vi "_PC_Daemon_RecipeEditor.vi"(5 "eng_mode_str":refnum<vi>, 8 "error in (no error)":errorcluster, 11 "Network\nstream":refnum<vi>) -> (0 "error out":errorcluster)   [LabVIEW 2018]
uses:
  System.Windows.Forms
  winForms/winForms editorType.ctl
  <vilib>/Utility/miscctls.llb/LVRowAndColumnTypeDef.ctl
  C:/ATI_MS_InstrumentControl/dll/ScintillaNET.dll
  dll/ScintillaNET.dll
  PublicSubVI/Ctl/RegistyFunc.ctl
  RecipeEditorPython/subVI/getScriptInfo.ctl
  PublicSubVI/Class/DataXML/DataXML dataType.ctl
  RecipeEditor/MSEncoder/MSEncoder.lvclass
  PublicSubVI/Class/QMH/QMH.lvclass
  PublicSubVI/Class/DataXML/DataXML.lvclass
panel:
  in  "SaveScript":bool
  in  "SaveScript_new":bool
  in  "open script":bool caption="OpenScript"
  in  "searchText":string
  in  "checkScript":bool
  in  "save_method":bool
  in  "applyScript":bool caption="apply_script"
  in  "help":bool caption="helpBtn"
  out "file path":string
  in  "script":refnum<k24>(container)
  in  "Parameter Tab":enum32{"User Parameter", "Instrument Parameter"}(tab)
  in  "user param table":string[][](table)
  in  "instr param table":string[][](table)
  in  "Dialogue":i32(listbox)=-1
  in  "stop":bool
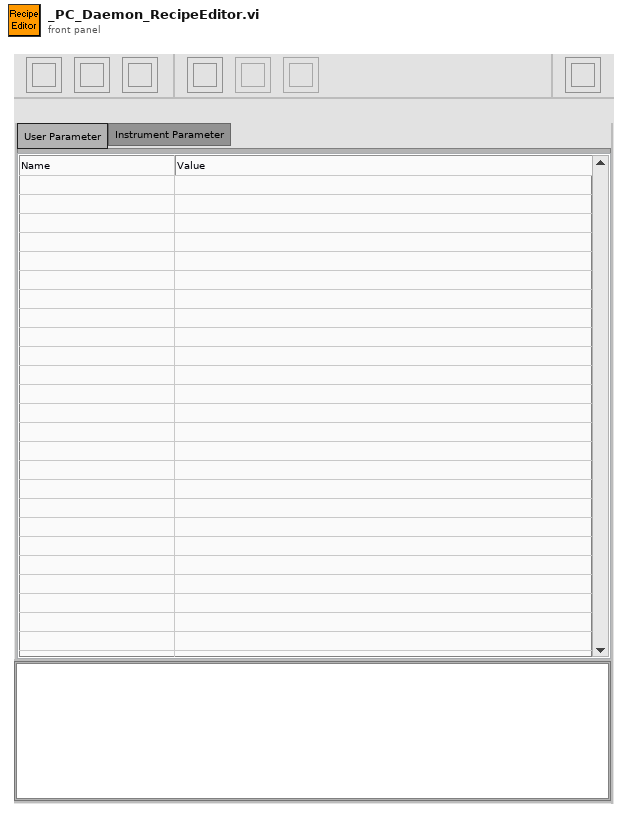
[diagram p1: front panel]
types:
  T1 = enum8{"Enabled", "Disabled", "Disabled and Grayed Out"}
  T2 = typedef "winForms editorType.ctl" = enum16{"Recipe", "SigProc", "Editor"}
  T3 = enum32{"Invalid", "Default", "Floating", "Floating/Auto-Hide", "Modal"}
  T4 = typedef "LVRowAndColumnTypeDef.ctl" = cluster{"Row":i32, "Column":i32}
  T5 = enum32{"Invalid", "Standard", "Closed", "Hidden", "Minimized", "Maximized"}
  T6 = enum16{"No Scaling", "Scale All Objects", "Scale Single Object"}
  T7 = typedef "LVRectTypeDef.ctl" = cluster{"Left":i16, "Top":i16, "Right":i16, "Bottom":i16}
  T8 = typedef "getScriptInfo.ctl" = enum16{"userEditor", "userParam", "instrParam", "sourcePath", "sourceTimeStamp", "versionInfo"}
  T9 = enum16{"open", "replace", "create", "open or create", "replace or create", "replace or create with confirmation"}
  T10 = typedef "DataXML dataType.ctl" = enum16{"Instrument", "UserInterface", "SampleType", "UserDefined"}
  T11 = cluster{"ProcessCodes":u64[], "WfmCodes":u64[], "Signal Remarks":cluster{"mzID":u64, "SignalInfo":cluster{"Label":string, "dt":dbl, "Length":u32, "RefVolt":dbl, "mzTable":cluster{"t":dbl[], "mz":dbl[], "beta":dbl[]}}[]}, "scriptCode":string}
  T12 = typedef "eventvkey.ctl" = enum16{"ASCII", "Enter", "Return", "Shift", "Ctrl", "Alt", "Cmd", "Opt", "Caps", "NumLock", "Clear", "Break", "Up", "Down", "Left", "Right", "Insert", "Delete", "Home", "End", "PageUp", "PageDown", "Escape", "Help", "Pause", "ScrollLock", "F1", "F2", "F3", "F4", "F5", "F6", "F7", "F8", "F9", "F10", "F11", "F12", "F13", "F14", "F15", "F16", "F17", "F18", "F19", "F20", "F21", "F22", "F23", "F24", "Play", "VolumeUp", "VolumeDown", "Mute", "Two Byte Char"}
  T13 = typedef "RegistyFunc.ctl" = enum16{"None", "FileAutoSave", "FileNoise", "FileSN", "ExeStatu", "WorkFolderPath", "MethodPath", "AVGItem", "LoopItem", "AutoRun", "BGColor", "LineColor", "LineWidth", "XGrid", "YGrid", "DeviceRefnum"}
  T14 = typedef "LVPoint32TypeDef.ctl" = cluster{"Horizontal":i32, "Vertical":i32}
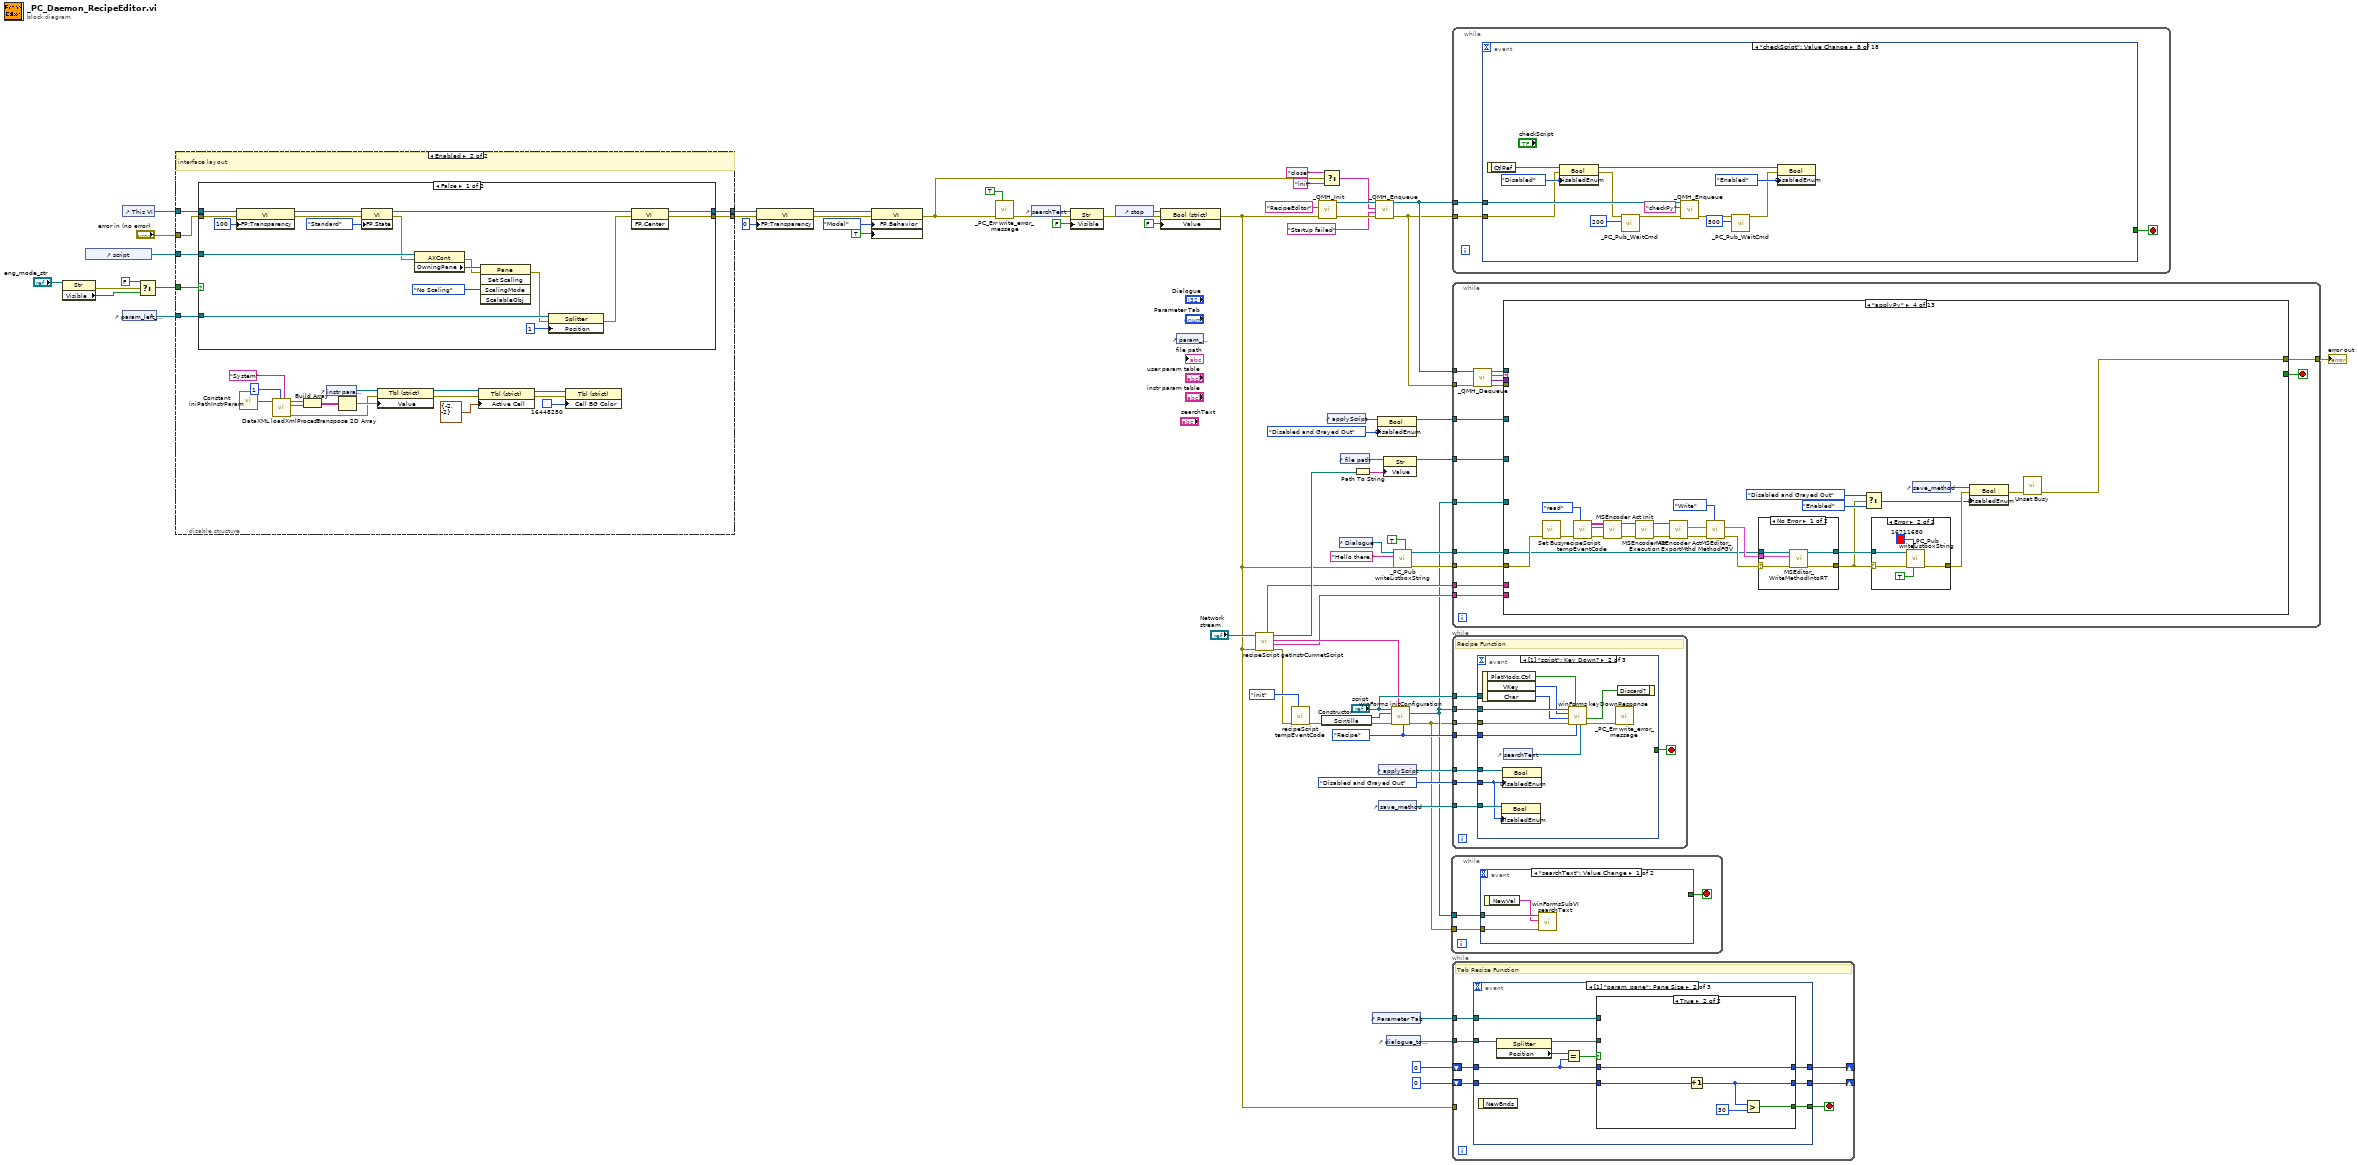
[diagram p0: block diagram]
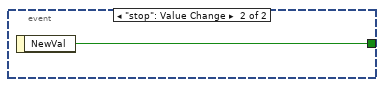
[diagram p2: hidden frame]
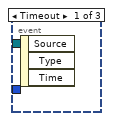
[diagram p3: hidden frame]
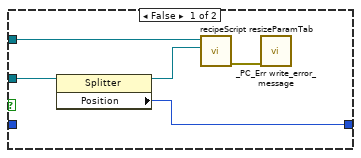
[diagram p4: hidden frame]
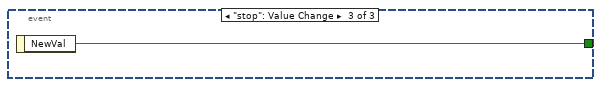
[diagram p5: hidden frame]
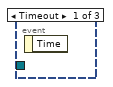
[diagram p6: hidden frame]
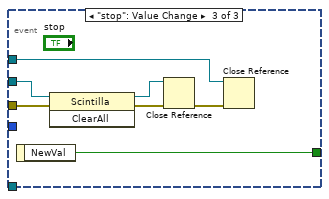
[diagram p7: hidden frame]
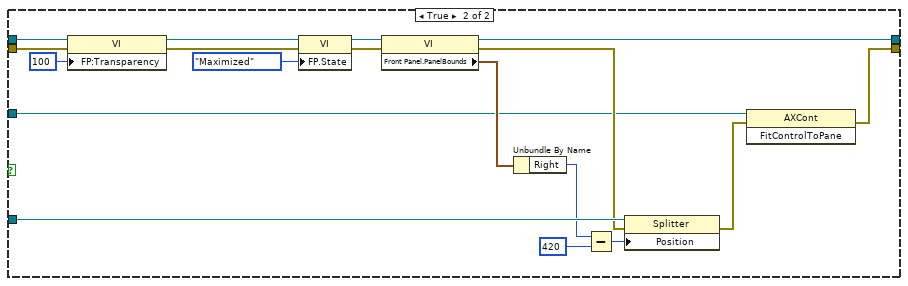
[diagram p9: hidden frame]
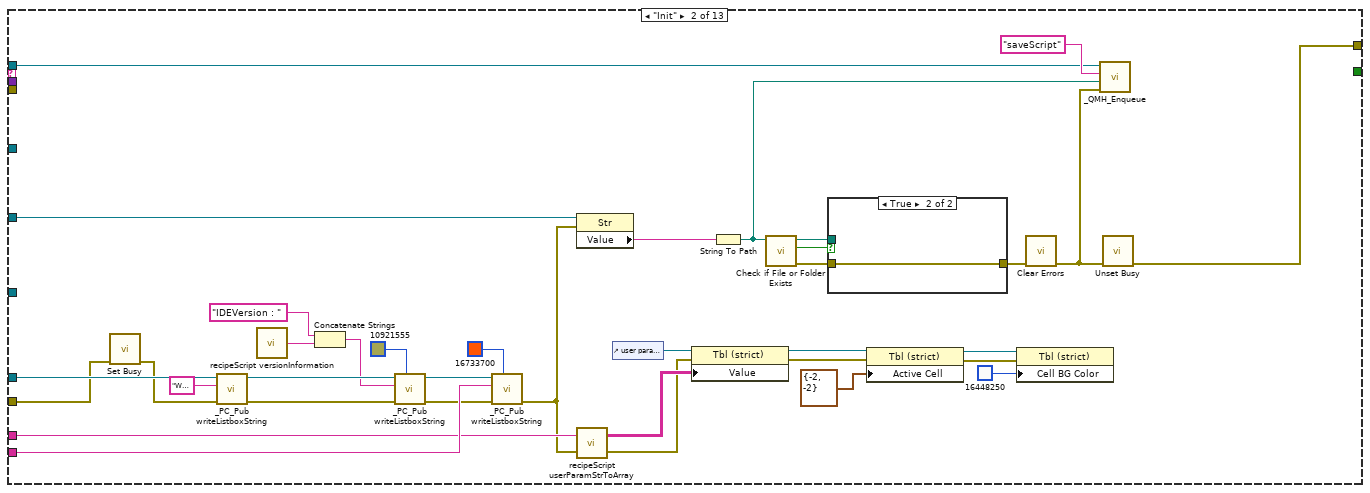
[diagram p11: hidden frame]
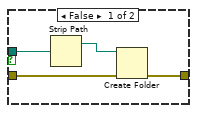
[diagram p12: hidden frame]
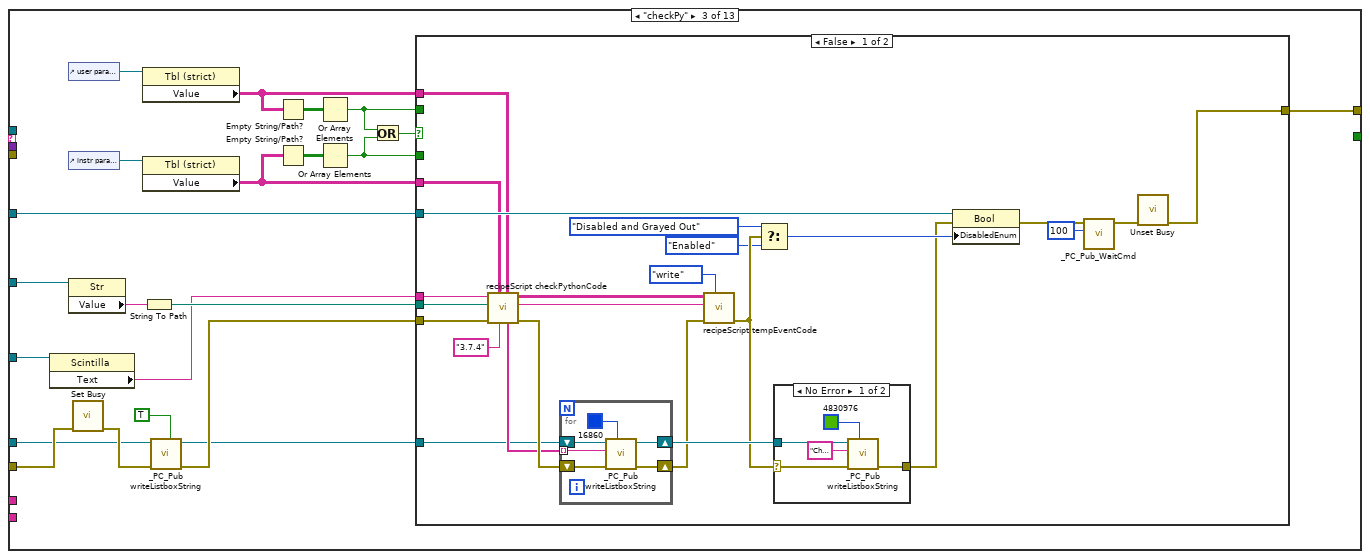
[diagram p13: hidden frame]
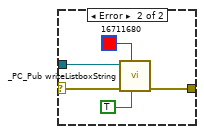
[diagram p14: hidden frame]
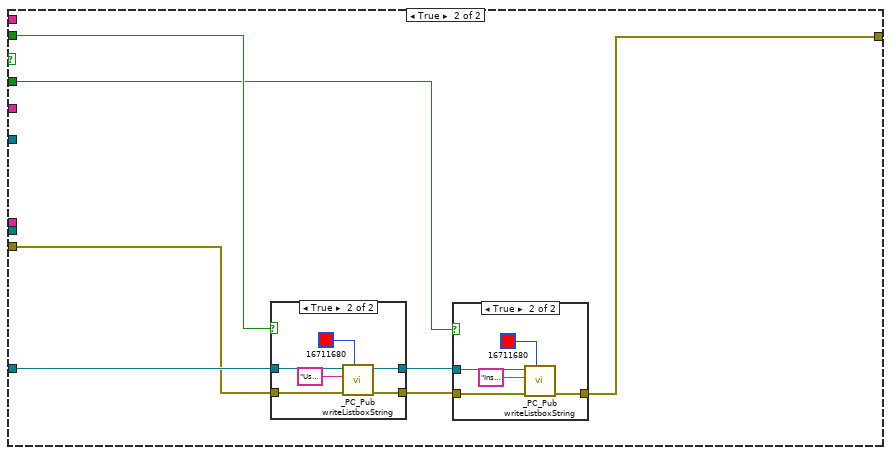
[diagram p15: hidden frame]
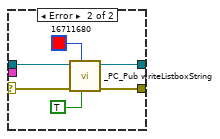
[diagram p19: hidden frame]
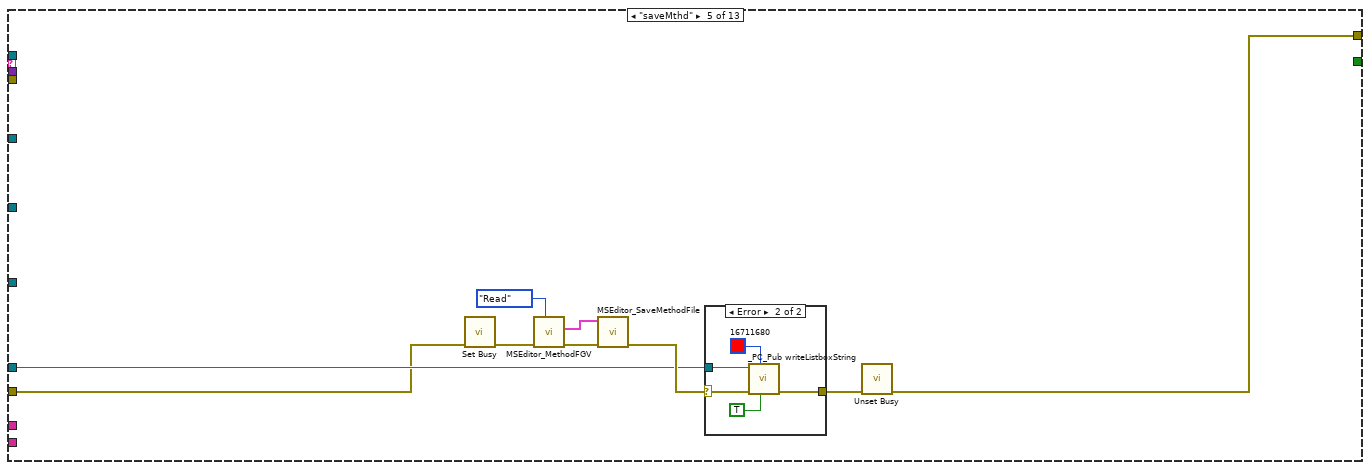
[diagram p20: hidden frame]
diagram:
  w15 = winForms_editorType."Recipe" ("editorType")
  n1 = property class="Str"(reference="eng_mode_str") -> (error out=w40:errorcluster, "Visible"=w39:bool)  [unwired: 1 in, 1 out]
  n2 = control-ref of="script"() -> (w36:refnum<vi>)
  n3 = control-ref of="param_left_spl"() -> (w64:refnum<vi>)
  n4 = control-ref of="This VI"() -> (w43:refnum<vi>)
  n5 = Select(t=FALSE, s=w40, f=w39) -> (s? t:f=w37:bool)
  n6 = disable-structure shown="Enabled" {
    disable-tunnel: w37 -> [_ w68]
    disable-tunnel: "error in (no error)" -> [_ w85]
    disable-tunnel: w43 -> [_ w87]
    disable-tunnel: [_ w86] -> w65
    disable-tunnel: w64 -> [_ w89]
    disable-tunnel: w36 -> [_ w88]
    disable-tunnel: [_ w69] -> w41
    frame Disabled {
    }
    frame Enabled {
      # "interface layout"
      n7 = case shown="False" w68 {
        tunnel: w89 -> [w107 w125]
        tunnel: w88 -> [w102 w114]
        tunnel: w87 -> [w99 w112]
        tunnel: [w90 w119] -> w86
        tunnel: [w91 w108] -> w69
        tunnel: w85 -> [w98 w111]
        frame False {
          n8 = property class="VI"(reference=w99, error in=w98, "FP:Transparency"=u8 100 ("Front Panel Window:Transparency")) -> (reference out=w96:refnum<vi>, error out=w95:errorcluster)
          n9 = property class="VI"(reference=w96, error in=w95, "FP.State"=T5."Standard" ("Front Panel Window:State")) -> (reference out=w93:refnum<vi>, error out=w94:errorcluster)
          n10 = property class="AXCont"(reference=w102, error in=w94) -> (error out=w103:errorcluster, "OwningPane"=w105:refnum<vi>)  [unwired: 1 out]
          n11 = invoke class="Pane" method="Set Scaling"(reference=w105, error in=w103, "ScalingMode"=T6."No Scaling" ("Scaling Mode")) -> (error out=w101:errorcluster)  [unwired: 2 in, 4 out]
          n12 = property class="Splitter"(reference=w107, error in=w101, "Position"=1 ("Splitter Position")) -> (error out=w92:errorcluster)  [unwired: 1 out]
          n13 = invoke class="VI" method="FP.Center"(reference=w93, error in=w92) -> (reference out=w90:refnum<vi>, error out=w91:errorcluster)  [unwired: 1 in, 1 out]
        }
        frame True {
          n14 = property class="VI"(reference=w112, error in=w111, "FP:Transparency"=u8 100 ("Front Panel Window:Transparency")) -> (reference out=w110:refnum<vi>, error out=w109:errorcluster)
          n15 = property class="VI"(reference=w110, error in=w109, "FP.State"=T5."Maximized" ("Front Panel Window:State")) -> (reference out=w122:refnum<vi>, error out=w121:errorcluster)
          n16 = property class="VI"(reference=w122, error in=w121) -> (reference out=w119:refnum<vi>, error out=w120:errorcluster, "Front Panel.PanelBounds"=w118:T7)
          n17 = Unbundle By Name(w118) -> ("Right"=w117:i16)
          n18 = Subtract(x=w117, y=i16 420) -> (x-y=w115:i16)
          n19 = property class="Splitter"(reference=w125, error in=w120, "Position"=w115) -> (error out=w124:errorcluster)  [unwired: 1 out]
          n20 = invoke class="AXCont" method="FitControlToPane"(reference=w114, error in=w124) -> (error out=w108:errorcluster)  [unwired: 1 in, 2 out]
        }
      }
      n21 = call "Constant iniPathInstrParam.vi"() -> ("appended path"=w81:path)
      n22 = call "DataXML loadXmlProcess.vi"("target name"="System", "level"=u8 1, "xml_data_path"=w81) -> ("error IO"=w70:errorcluster, "value"=w83:string[], "name"=w82:string[])  [unwired: 5 in, 1 out]
      n23 = Build Array(w82, w83) -> (w84:string[][])
      n24 = control-ref of="instr param table"() -> (w74:refnum<vi>)
      n25 = Transpose 2D Array(2D array=w84) -> (transposed array=w73:string[][])
      n26 = property class="Tbl (strict)"(reference=w74, error in=w70, "Value"=w73) -> (reference out=w75:refnum<vi>, error out=w76:errorcluster)
      n27 = property class="Tbl (strict)"(reference=w75, error in=w76, "Active Cell"=T4 {"Row"=-2, "Column"=-2} ("Active Cell:Active Cell")) -> (reference out=w77:refnum<vi>, error out=w78:errorcluster)
      n28 = property class="Tbl (strict)"(reference=w77, error in=w78, "Cell BG Color"=u32 16448250) -> ()  [unwired: 2 out]
    }
  }
  n29 = property class="VI"(reference=w65, error in=w41, "FP:Transparency"=u8 0 ("Front Panel Window:Transparency")) -> (reference out=w57:refnum<vi>, error out=w58:errorcluster)
  n30 = property class="VI"(reference=w57, error in=w58, "FP.Behavior"=T3."Modal" ("Front Panel Window:Behavior"), "Front Panel.IsFrontmost"=TRUE ("Front Panel Window:Is Frontmost")) -> (error out=w28:errorcluster)  [unwired: 1 out]
  n31 = call "_PC_Err write_error_message.vi"("show msg( T )"=TRUE, "error in"=w28) -> ("error out"=w5:errorcluster)  [unwired: 9 in]
  n32 = control-ref of="searchText"() -> (w6:refnum<vi>)
  n33 = property class="Str"(reference=w6, error in=w5, "Visible"=FALSE) -> (error out=w4:errorcluster)  [unwired: 1 out]
  n34 = control-ref of="stop"() -> (w35:refnum<vi>)
  n35 = property class="Bool (strict)"(reference=w35, error in=w4, "Value"=FALSE) -> (error out=w17:errorcluster)  [unwired: 1 out]
  n36 = control-ref of="param_pane"() -> ()  [unwired: 1 out]
  n37 = call "recipeScript getInstrCurrnetScript.vi"("error in (no error)"=w17, "Network\nstream"="Network\nstream") -> ("error out"=w13:errorcluster, "versionInfo"=w8:string, "initScriptCode"=w16:string, "initFilePath"=w19:path, "userParam"=w7:string)  [unwired: 5 in]
  n38 = call "recipeScript tempEventCode.vi"("type"=enum16{"init", "write", "read"}."init", "error in (no error)"=w13) -> ("error out"=w12:errorcluster)  [unwired: 7 in, 2 out]
  n39 = call "_QMH_Init.vi"("error in (no error)"=w17, "name (unnamed)"="RecipeEditor") -> ("error out"=w62:errorcluster, "QMH out"=w63:refnum<class "QMH.lvclass">)  [unwired: 8 in]
  n40 = constructor class="Scintilla"(error in=w12) -> (reference out=w25:refnum<k24>, error out=w24:errorcluster)  [unwired: 2 in, 1 out]
  n41 = Select(t="close" ("Msg"), s=w28, f="init" ("Msg")) -> (s? t:f=w51:string)
  n42 = control-ref of="applyScript"() -> (w46:refnum<vi>)
  n43 = control-ref of="Dialogue"() -> (w55:refnum<vi>)
  n44 = control-ref of="file path"() -> (w21:refnum<vi>)
  n45 = Path To String(path=w19) -> (string=w18:string)
  n46 = control-ref of="Parameter Tab"() -> (w32:refnum<vi>)
  n47 = call "_QMH_Enqueue.vi"("error in (no error)"=w62, "Data"="Startup failed", "Msg"=w51, "QMH in"=w63) -> ("error out"=w48:errorcluster, "QMH out"=w61:refnum<class "QMH.lvclass">)  [unwired: 6 in]
  n48 = property class="Bool"(reference=w46, "DisabledEnum"=T1."Disabled and Grayed Out" ("Disabled")) -> (reference out=w45:refnum<vi>)  [unwired: 1 in, 1 out]
  n49 = control-ref of="applyScript"() -> (w11:refnum<vi>)
  n50 = control-ref of="save_method"() -> (w9:refnum<vi>)
  n51 = property class="Str"(reference=w21, "Value"=w18) -> (reference out=w20:refnum<vi>)  [unwired: 1 in, 1 out]
  n52 = control-ref of="dialogue_top_spl"() -> (w31:refnum<vi>)
  n53 = call "winForms initConfiguration.vi"("editorType"=w15, "initText"=w16, "error in (no error)"=w24, "scintillaRefNum in"=w25, "panelRefNum"="script") -> ("error out"=w1:errorcluster, "scintillaRefNum out"=w2:refnum<k24>)  [unwired: 5 in]
  n54 = call "_PC_Pub writeListboxString.vi"("Reset (F)"=TRUE ("Reset"), "error in (no error)"=w17, "update_Str"="Hello there." ("New string"), "Listbox Ref Input"=w55) -> ("error out"=w26:errorcluster, "Listbox Ref Output"=w27:refnum<vi>)  [unwired: 6 in]
  n55 = while {
    tunnel: w2 -> [w128]
    tunnel: w1 -> [w127]
    stop <- w126 stop-if-true
    n56 = event shown="[0] \"searchText\": Value Change" {
      selector: _ -> [_ _]
      dyn-events: _ -> [_ _]
      timeout: _ -> [_ _]
      tunnel: w128 -> [w131 _]
      tunnel: w127 -> [w130 _]
      tunnel: [_ w132] -> w126
      event "searchText": Value Change {
        n57 = event-data() -> ("NewVal"=w129:string)  [unwired: 1 in]
        n58 = call "winFormsSubVI searchText.vi"("error in (no error)"=w130, "searchString"=w129, "scintillaRefNum in"=w131) -> ()  [unwired: 7 in, 2 out]
      }
      event "stop": Value Change {
        n59 = event-data() -> ("NewVal"=w132:bool)  [unwired: 1 in]
      }
    }
  }
  n60 = while {
    tunnel: w61 -> [w147]
    tunnel: w48 -> [w146]
    tunnel: [w143] -> w49
    tunnel: w20 -> [w141]
    tunnel: w27 -> [w140]
    tunnel: w26 -> [w139]
    tunnel: w45 -> [w138]
    tunnel: w2 -> [w136]
    tunnel: w8 -> [w134]
    tunnel: w7 -> [w133]
    stop <- w142 stop-if-true
    n61 = call "_QMH_Dequeue.vi"("error in (no error)"=w146, "QMH in"=w147) -> ("error out"=w135:errorcluster, "Data"=w144:variant, "Msg"=w145:string, "QMH out"=w137:refnum<class "QMH.lvclass">)  [unwired: 4 in, 2 out]
    n62 = case shown="\"applyPy\"" w145 {
      tunnel: w144 -> [_ _ _ _ _ w339 w408 _ _ w472 _ _ w554]
      tunnel: [_ w180 w197 w296 w314 w340 w410 _ w456 w460 w497 _ w555] -> w143
      tunnel: [_ _ _ _ _ _ _ _ _ _ _ _ TRUE] -> w142
      tunnel: w141 -> [_ w179 w207 _ _ w335 w404 _ _ _ _ _ _]
      tunnel: w140 -> [_ w183 w200 w280 w318 w331 w402 _ _ _ _ _ _]
      tunnel: w139 -> [_ w182 w203 w295 w317 w342 w403 _ w457 w471 w499 w538 w540]
      tunnel: w138 -> [_ _ w202 _ _ _ _ _ _ _ _ _ _]
      tunnel: w137 -> [_ w172 _ _ _ _ _ _ _ _ _ _ _]
      tunnel: w136 -> [_ _ w206 _ _ w343 w401 _ _ _ _ _ _]
      tunnel: w135 -> [_ _ _ _ _ _ _ _ _ _ _ _ _]
      tunnel: w134 -> [_ w168 _ _ _ _ _ _ _ _ _ _ _]
      tunnel: w133 -> [_ w159 _ _ _ _ _ _ _ _ _ _ _]
      frame Default {
      }
      frame "Init" {
        n63 = call <vilib>:"Set Busy.vi"("error in (no error)"=w182) -> ("error out"=w181:errorcluster)  [unwired: 9 in, 1 out]
        n64 = call "_PC_Pub writeListboxString.vi"("error in (no error)"=w181, "update_Str"="Welcome to use AcroMass MS script editor." ("New string"), "Listbox Ref Input"=w183) -> ("error out"=w153:errorcluster, "Listbox Ref Output"=w154:refnum<vi>)  [unwired: 7 in]
        n65 = call "recipeScript versionInformation.vi"() -> ("verInfo"=w149:string)
        n66 = Concatenate Strings("IDEVersion : ", w149) -> (w148:string)
        n67 = call "_PC_Pub writeListboxString.vi"("String Color"=u32 10921555, "error in (no error)"=w153, "update_Str"=w148, "Listbox Ref Input"=w154) -> ("error out"=w151:errorcluster, "Listbox Ref Output"=w152:refnum<vi>)  [unwired: 6 in]
        n68 = call "_PC_Pub writeListboxString.vi"("String Color"=u32 16733700, "error in (no error)"=w151, "update_Str"=w168, "Listbox Ref Input"=w152) -> ("error out"=w158:errorcluster)  [unwired: 6 in, 1 out]
        n69 = property class="Str"(reference=w179, error in=w158) -> ("Value"=w178:string)  [unwired: 2 out]
        n70 = call "recipeScript userParamStrToArray.vi"("error in (no error)"=w158, "recipeScript"=w159) -> ("error out"=w156:errorcluster, "userParam"=w157:string[][])
        n71 = control-ref of="user param table"() -> (w160:refnum<vi>)
        n72 = property class="Tbl (strict)"(reference=w160, error in=w156, "Value"=w157) -> (reference out=w163:refnum<vi>, error out=w164:errorcluster)
        n73 = String To Path(string=w178) -> (path=w170:path)
        n74 = call <vilib>:"Check if File or Folder Exists.vi"("path"=w170) -> ("error out"=w175:errorcluster, "file or folder exists?"=w177:bool, "dup path"=w176:path)  [unwired: 8 in]
        n75 = case shown="True" w177 {
          tunnel: w176 -> [w187 _]
          tunnel: w175 -> [w185 w188]
          tunnel: [w184 w188] -> w174
          frame False {
            n76 = Strip Path(path=w187) -> (stripped path=w186:path)  [unwired: 1 out]
            n77 = Create Folder(path (use dialog)=w186, error in=w185) -> (error out=w184:errorcluster)  [unwired: 1 in, 2 out]
          }
          frame True {
          }
        }
        n78 = property class="Tbl (strict)"(reference=w163, error in=w164, "Active Cell"=T4 {"Row"=-2, "Column"=-2} ("Active Cell:Active Cell")) -> (reference out=w165:refnum<vi>, error out=w166:errorcluster)
        n79 = property class="Tbl (strict)"(reference=w165, error in=w166, "Cell BG Color"=u32 16448250) -> ()  [unwired: 2 out]
        n80 = call <vilib>:"Clear Errors.vi"("error in (no error)"=w174) -> ("error out"=w171:errorcluster)  [unwired: 5 in, 1 out]
        n81 = call "_QMH_Enqueue.vi"("error in (no error)"=w171, "Data"=w170, "Msg"="saveScript", "QMH in"=w172) -> ()  [unwired: 6 in, 2 out]
        n82 = call <vilib>:"Unset Busy.vi"("error in (no error)"=w171) -> ("error out"=w180:errorcluster)  [unwired: 10 in]
      }
      frame "checkPy" {
        n83 = property class="Scintilla"(reference=w206) -> ("Text"=w204:string)  [unwired: 1 in, 2 out]
        n84 = control-ref of="user param table"() -> (w209:refnum<vi>)
        n85 = control-ref of="instr param table"() -> (w210:refnum<vi>)
        n86 = property class="Str"(reference=w207) -> ("Value"=w208:string)  [unwired: 1 in, 2 out]
        n87 = call <vilib>:"Set Busy.vi"("error in (no error)"=w203) -> ("error out"=w201:errorcluster)  [unwired: 9 in, 1 out]
        n88 = property class="Tbl (strict)"(reference=w209) -> ("Value"=w194:string[][])  [unwired: 1 in, 2 out]
        n89 = property class="Tbl (strict)"(reference=w210) -> ("Value"=w192:string[][])  [unwired: 1 in, 2 out]
        n90 = String To Path(string=w208) -> (path=w205:path)
        n91 = call "_PC_Pub writeListboxString.vi"("Reset (F)"=TRUE, "error in (no error)"=w201, "Listbox Ref Input"=w200) -> ("error out"=w198:errorcluster, "Listbox Ref Output"=w196:refnum<vi>)  [unwired: 7 in]
        n92 = Empty String/Path?(string/path=w194) -> (empty?=w195:bool[][])
        n93 = Empty String/Path?(string/path=w192) -> (empty?=w193:bool[][])
        n94 = Or Array Elements(Boolean array=w195) -> (logical OR=w190:bool)
        n95 = Or Array Elements(Boolean array=w193) -> (logical OR=w189:bool)
        n96 = Or(x=w190, y=w189) -> (x .or. y?=w191:bool)
        n97 = case shown="False" w191 {
          tunnel: w205 -> [w234 _]
          tunnel: w204 -> [w233 _]
          tunnel: w202 -> [w224 _]
          tunnel: w198 -> [w218 w255]
          tunnel: [w214 w251] -> w197
          tunnel: w196 -> [w213 w256]
          tunnel: w194 -> [w212 _]
          tunnel: w192 -> [w211 _]
          tunnel: w190 -> [_ w257]
          tunnel: w189 -> [_ w254]
          frame False {
            n98 = call "recipeScript checkPythonCode.vi"("userTable"=w212, "Python version(3.7.4)"="3.7.4" ("Python version"), "instrTable"=w211, "error in (no error)"=w218, "sourceFilePath"=w234, "recipeScript"=w233) -> ("error out"=w228:errorcluster, "scriptPythonCode"=w230:string, "eventProcess"=w231:string[][], "showMsg"=w227:string[])  [unwired: 2 in]
            n99 = for {
              tunnel: w227 -> [w237] mode=indexing
              shift-right: [w238] -> w226
              shift-left: w213 -> [w239]
              shift-right: [w235] -> w225
              shift-left: w228 -> [w236]
              n100 = call "_PC_Pub writeListboxString.vi"("String Color"=u32 16860, "error in (no error)"=w236, "update_Str"=w237, "Listbox Ref Input"=w239) -> ("error out"=w235:errorcluster, "Listbox Ref Output"=w238:refnum<vi>)  [unwired: 6 in]
            }
            n101 = call "recipeScript tempEventCode.vi"("type"=enum16{"init", "write", "read"}."write", "error in (no error)"=w225, "scriptPythonCode in"=w230, "eventProcess in"=w231) -> ("error out"=w223:errorcluster)  [unwired: 5 in, 2 out]
            n102 = Select(t=T1."Disabled and Grayed Out" ("Disabled"), s=w223, f=T1."Enabled" ("Disabled")) -> (s? t:f=w220:T1)
            n103 = case shown="No Error" w223 {
              selector: w223 -> [w244 w247]
              tunnel: w226 -> [w245 w248]
              tunnel: [w243 w246] -> w219
              frame No Error {
                n104 = call "_PC_Pub writeListboxString.vi"("String Color"=u32 4830976, "error in (no error)"=w244, "update_Str"="Check Pass...", "Listbox Ref Input"=w245) -> ("error out"=w243:errorcluster)  [unwired: 6 in, 1 out]
              }
              frame Error {
                n105 = call "_PC_Pub writeListboxString.vi"("Display Error Msg? (F)"=TRUE ("Display Error Msg? (T)"), "String Color"=u32 16711680, "error in (no error)"=w247, "Listbox Ref Input"=w248) -> ("error out"=w246:errorcluster)  [unwired: 6 in, 1 out]
              }
            }
            n106 = property class="Bool"(reference=w224, error in=w219, "DisabledEnum"=w220) -> (error out=w217:errorcluster)  [unwired: 1 out]
            n107 = call "_PC_Pub_WaitCmd.vi"("milliseconds to wait"=u32 100, "error in (no error)"=w217) -> ("error out"=w215:errorcluster)  [unwired: 9 in]
            n108 = call <vilib>:"Unset Busy.vi"("error in (no error)"=w215) -> ("error out"=w214:errorcluster)  [unwired: 10 in]
          }
          frame True {
            n109 = case shown="True" w257 {
              tunnel: w256 -> [w265 w270]
              tunnel: w255 -> [w264 w269]
              tunnel: [w265 w267] -> w253
              tunnel: [w264 w266] -> w252
              frame False {
              }
              frame True {
                n110 = call "_PC_Pub writeListboxString.vi"("String Color"=u32 16711680, "error in (no error)"=w269, "update_Str"="User parameter contains characters not allowed.", "Listbox Ref Input"=w270) -> ("error out"=w266:errorcluster, "Listbox Ref Output"=w267:refnum<vi>)  [unwired: 6 in]
              }
            }
            n111 = case shown="True" w254 {
              tunnel: w253 -> [_ w262]
              tunnel: w252 -> [w258 w261]
              tunnel: [w258 w259] -> w251
              frame False {
              }
              frame True {
                n112 = call "_PC_Pub writeListboxString.vi"("String Color"=u32 16711680, "error in (no error)"=w261, "update_Str"="Instrument parameter contains characters not allowed.", "Listbox Ref Input"=w262) -> ("error out"=w259:errorcluster)  [unwired: 6 in, 1 out]
              }
            }
          }
        }
      }
      frame "applyPy" {
        n113 = call <vilib>:"Set Busy.vi"("error in (no error)"=w295) -> ("error out"=w279:errorcluster)  [unwired: 9 in, 1 out]
        n114 = call "recipeScript tempEventCode.vi"("type"=enum16{"init", "write", "read"}."read", "error in (no error)"=w279) -> ("error out"=w278:errorcluster, "scriptPythonCode out"=w276:string, "eventProcess out"=w277:string[][])  [unwired: 7 in]
        n115 = call "MSEncoder Act Init.vi"("error in (no error)"=w278, "scriptPythonCode"=w276, "eventProcess"=w277) -> ("error out"=w293:errorcluster, "MSEncoder out"=w294:refnum<class "MSEncoder.lvclass">)  [unwired: 5 in]
        n116 = call-dynamic "MSEncoder Act Execution.vi"("error in (no error)"=w293, "MSEncoder in"=w294) -> ("error out"=w291:errorcluster, "MSEncoder out"=w292:refnum<class "MSEncoder.lvclass">)  [unwired: 8 in]
        n117 = call-dynamic "MSEncoder Act ExportMthd.vi"("error in (no error)"=w291, "MSEncoder in"=w292) -> ("error out"=w288:errorcluster, "Mthd out"=w289:T11)  [unwired: 8 in]
        n118 = call "MSEditor_MethodFGV.vi"("Mthd in"=w289, "error in (no error)"=w288, "Function"=enum16{"Write", "Read"}."Write") -> ("Mthd out"=w286:T11, "error out"=w287:errorcluster)  [unwired: 6 in]
        n119 = case shown="No Error" w287 {
          selector: w287 -> [w306 w310]
          tunnel: w280 -> [w307 w311]
          tunnel: [w304 w309] -> w273
          tunnel: w286 -> [w305 _]
          tunnel: [w303 w308] -> w285
          frame No Error {
            n120 = call "MSEditor_WriteMethodIntoRT.vi"("error in"=w306, "Mthd in"=w305, "listbox ref in"=w307) -> ("error out"=w304:errorcluster, "listbox ref out"=w303:refnum<vi>)  [unwired: 7 in]
          }
          frame Error {
            n121 = call "_PC_Pub writeListboxString.vi"("Display Error Msg? (F)"=TRUE ("Display Error Msg? (T)"), "String Color"=u32 16711680, "error in (no error)"=w310, "Listbox Ref Input"=w311) -> ("error out"=w309:errorcluster, "Listbox Ref Output"=w308:refnum<vi>)  [unwired: 6 in]
          }
        }
        n122 = Select(t=T1."Disabled and Grayed Out" ("Disabled"), s=w273, f=T1."Enabled" ("Disabled")) -> (s? t:f=w272:T1)
        n123 = case shown="Error" w273 {
          selector: w273 -> [w297 w299]
          tunnel: w285 -> [_ w300]
          tunnel: [w297 w298] -> w283
          frame No Error {
          }
          frame Error {
            n124 = call "_PC_Pub writeListboxString.vi"("Display Error Msg? (F)"=TRUE ("Display Error Msg? (T)"), "String Color"=u32 16711680, "error in (no error)"=w299, "Listbox Ref Input"=w300) -> ("error out"=w298:errorcluster)  [unwired: 6 in, 1 out]
          }
        }
        n125 = control-ref of="save_method"() -> (w284:refnum<vi>)
        n126 = property class="Bool"(reference=w284, error in=w283, "DisabledEnum"=w272) -> (error out=w282:errorcluster)  [unwired: 1 out]
        n127 = call <vilib>:"Unset Busy.vi"("error in (no error)"=w282) -> ("error out"=w296:errorcluster)  [unwired: 10 in]
      }
      frame "saveMthd" {
        n128 = call <vilib>:"Set Busy.vi"("error in (no error)"=w317) -> ("error out"=w316:errorcluster)  [unwired: 9 in, 1 out]
        n129 = call "MSEditor_MethodFGV.vi"("error in (no error)"=w316, "Function"=enum16{"Write", "Read"}."Read") -> ("Mthd out"=w320:T11, "error out"=w321:errorcluster)  [unwired: 7 in]
        n130 = call "MSEditor_SaveMethodFile.vi"("error in (no error)"=w321, "Mthd in"=w320) -> ("error out"=w319:errorcluster)  [unwired: 9 in]
        n131 = case shown="Error" w319 {
          selector: w319 -> [w323 w325]
          tunnel: w318 -> [_ w326]
          tunnel: [w323 w324] -> w315
          frame No Error {
          }
          frame Error {
            n132 = call "_PC_Pub writeListboxString.vi"("Display Error Msg? (F)"=TRUE ("Display Error Msg? (T)"), "String Color"=u32 16711680, "error in (no error)"=w325, "Listbox Ref Input"=w326) -> ("error out"=w324:errorcluster)  [unwired: 6 in, 1 out]
          }
        }
        n133 = call <vilib>:"Unset Busy.vi"("error in (no error)"=w315) -> ("error out"=w314:errorcluster)  [unwired: 10 in]
      }
      frame "openFile" {
        n134 = call <vilib>:"Set Busy.vi"("error in (no error)"=w342) -> ("error out"=w337:errorcluster)  [unwired: 9 in, 1 out]
        n135 = Variant To Data(error in=w337, type=path "" ("selected path"), Variant=w339) -> (data=w332:path, error out=w336:errorcluster)
        n136 = call "recipeScript setNewFilePath.vi"("newfilePath"=w332, "error in (no error)"=w336, "filePathRefnum in"=w335) -> ("error out"=w333:errorcluster, "valid"=w334:bool)  [unwired: 6 in, 1 out]
        n137 = case shown="True" w334 {
          tunnel: w343 -> [_ w382]
          tunnel: w333 -> [w349 w372]
          tunnel: w332 -> [_ w373]
          tunnel: w331 -> [w350 w363]
          tunnel: [w345 w370] -> w330
          tunnel: [w344 w366] -> w329
          frame False {
            n138 = call "_PC_Pub writeListboxString.vi"("Display Error Msg? (F)"=TRUE ("Display Error Msg? (T)"), "String Color"=u32 16711680, "error in (no error)"=w349, "update_Str"="Invalid path" ("message"), "Listbox Ref Input"=w350) -> ("error out"=w345:errorcluster, "Listbox Ref Output"=w344:refnum<vi>)  [unwired: 5 in]
          }
          frame True {
            n139 = call "_PC_Pub writeListboxString.vi"("Reset (F)"=TRUE, "Listbox Ref Input"=w363) -> ("error out"=w357:errorcluster, "Listbox Ref Output"=w358:refnum<vi>)  [unwired: 8 in]
            n140 = Open/Create/Replace File(file path (use dialog)=w373, error in=w372, operation (0:open)=T9."open", access (0:read/write)=enum16{"read/write", "read-only", "write-only"}."read-only") -> (refnum out=w381:refnum<file>, error out=w380:errorcluster)  [unwired: 2 in, 1 out]
            n141 = Read from Binary File(5:"", 8:w380, 11:w381) -> (0:w378:errorcluster, 2:w353:string, 3:w379:refnum<file>)  [unwired: 3 in, 1 out]
            n142 = call "recipeScript versionInformation.vi"() -> ("verInfo"=w361:string)
            n143 = Close File(refnum=w379, error in=w378) -> (error out=w374:errorcluster)  [unwired: 1 out]
            n144 = Concatenate Strings("IDEVersion : ", w361) -> (w362:string)
            n145 = call "recipeScript getScriptInfo.vi"("sysCode"=w353, "method"=getScriptInfo."userEditor") -> ("output"=w352:string)  [unwired: 1 in]
            n146 = call "recipeScript getScriptInfo.vi"("sysCode"=w353, "method"=getScriptInfo."versionInfo") -> ("output"=w365:string)  [unwired: 1 in]
            n147 = call "_PC_Pub writeListboxString.vi"("String Color"=u32 10921555, "error in (no error)"=w357, "update_Str"=w362, "Listbox Ref Input"=w358) -> ("error out"=w355:errorcluster, "Listbox Ref Output"=w356:refnum<vi>)  [unwired: 6 in]
            n148 = Empty String/Path?(string/path=w352) -> (empty?=w354:bool)
            n149 = Select(t=w353, s=w354, f=w352) -> (s? t:f=w351:string)
            n150 = property class="Scintilla"(reference=w382, error in=w374, "Text"=w351) -> (error out=w370:errorcluster)  [unwired: 1 out]
            n151 = call "_PC_Pub writeListboxString.vi"("String Color"=u32 16733700, "error in (no error)"=w355, "update_Str"=w365, "Listbox Ref Input"=w356) -> ("Listbox Ref Output"=w366:refnum<vi>)  [unwired: 6 in, 1 out]
            n152 = call "_PC_Err write_error_message.vi"("show msg( T )"=FALSE ("skipWrong( T )"), "error in"=w370) -> ()  [unwired: 9 in, 1 out]
          }
        }
        n153 = case shown="Error" w330 {
          selector: w330 -> [w383 w385]
          tunnel: w329 -> [_ w386]
          tunnel: [w383 w384] -> w341
          frame No Error {
          }
          frame Error {
            n154 = call "_PC_Pub writeListboxString.vi"("Display Error Msg? (F)"=TRUE ("Display Error Msg? (T)"), "String Color"=u32 16711680, "error in (no error)"=w385, "Listbox Ref Input"=w386) -> ("error out"=w384:errorcluster)  [unwired: 6 in, 1 out]
          }
        }
        n155 = call <vilib>:"Unset Busy.vi"("error in (no error)"=w341) -> ("error out"=w340:errorcluster)  [unwired: 10 in]
      }
      frame "saveScript" {
        n156 = call <vilib>:"Set Busy.vi"("error in (no error)"=w403) -> ("error out"=w407:errorcluster)  [unwired: 9 in, 1 out]
        n157 = Variant To Data(error in=w407, type=path "" ("selected path"), Variant=w408) -> (data=w405:path, error out=w406:errorcluster)
        n158 = case shown="No Error" w406 {
          tunnel: w405 -> [w439 _]
          tunnel: w404 -> [w438 w444]
          tunnel: [w439 w442] -> w396
          tunnel: [_ w441] -> w395
          tunnel: [w438 w440] -> w389
          frame No Error {
          }
          frame Error {
            n159 = property class="Str"(reference=w444) -> (reference out=w440:refnum<vi>, error out=w441:errorcluster, "Value"=w443:string)  [unwired: 1 in]
            n160 = String To Path(string=w443) -> (path=w442:path)
          }
        }
        n161 = property class="Scintilla"(reference=w401) -> (error out=w398:errorcluster, "Text"=w397:string)  [unwired: 1 in, 1 out]
        n162 = call "recipeScript repeatFile.vi"("error in (no error)"=w395, "path"=w396) -> ("error out"=w394:errorcluster, "dup path"=w393:path)  [unwired: 8 in]
        n163 = control-ref of="user param table"() -> (w399:refnum<vi>)
        n164 = control-ref of="instr param table"() -> (w400:refnum<vi>)
        n165 = Empty String/Path?(string/path=w393) -> (empty?=w392:bool)
        n166 = case shown="False" w392 {
          tunnel: w400 -> [w425 _]
          tunnel: w399 -> [w424 _]
          tunnel: w398 -> [w421 _]
          tunnel: w397 -> [w420 _]
          tunnel: w394 -> [w419 w437]
          tunnel: w393 -> [w418 _]
          tunnel: [w415 w437] -> w390
          tunnel: w389 -> [w417 _]
          frame False {
            n167 = property class="Tbl (strict)"(reference=w424) -> (error out=w428:errorcluster, "Value"=w427:string[][])  [unwired: 1 in, 1 out]
            n168 = property class="Tbl (strict)"(reference=w425) -> (error out=w429:errorcluster, "Value"=w426:string[][])  [unwired: 1 in, 1 out]
            n169 = Merge Errors(w428, w429, w419, w421) -> (w414:errorcluster)
            n170 = Open/Create/Replace File(file path (use dialog)=w418, error in=w414, operation (0:open)=T9."replace or create", access (0:read/write)=enum16{"read/write", "read-only", "write-only"}."write-only") -> (refnum out=w430:refnum<file>, error out=w413:errorcluster)  [unwired: 2 in, 1 out]
            n171 = call "recipeScript generatePyScript.vi"("userTable"=w427, "instrTable"=w426, "error in (no error)"=w413, "recipeScript"=w420, "sourceFilePath"=w418) -> ("error out"=w412:errorcluster, "PyCode"=w433:string)  [unwired: 5 in]
            n172 = Write to Binary File(file (use dialog)=w430, data=w433, error in=w412) -> (refnum out=w432:refnum<file>, error out=w431:errorcluster)  [unwired: 3 in, 1 out]
            n173 = Close File(refnum=w432, error in=w431) -> (path=w416:path, error out=w415:errorcluster)
            n174 = case shown="No Error" w415 {
              tunnel: w417 -> [w435 _]
              tunnel: w416 -> [w434 _]
              frame No Error {
                n175 = Path To String(path=w434) -> (string=w436:string)
                n176 = property class="Str"(reference=w435, "Value"=w436) -> ()  [unwired: 1 in, 2 out]
              }
              frame Error {
              }
            }
          }
          frame True {
          }
        }
        n177 = case shown="Error" w390 {
          selector: w390 -> [w445 w447]
          tunnel: w402 -> [_ w448]
          tunnel: [w445 w446] -> w411
          frame No Error {
          }
          frame Error {
            n178 = call "_PC_Pub writeListboxString.vi"("Display Error Msg? (F)"=TRUE ("Display Error Msg? (T)"), "String Color"=u32 16711680, "error in (no error)"=w447, "Listbox Ref Input"=w448) -> ("error out"=w446:errorcluster)  [unwired: 6 in, 1 out]
          }
        }
        n179 = call "_PC_Err write_error_message.vi"("show msg( T )"=FALSE ("skipWrong( T )"), "error in"=w390) -> ()  [unwired: 9 in, 1 out]
        n180 = call <vilib>:"Unset Busy.vi"("error in (no error)"=w411) -> ("error out"=w410:errorcluster)  [unwired: 10 in]
      }
      frame "userParamUpd" {
      }
      frame "instrParamUpd" {
        n181 = call <vilib>:"Set Busy.vi"("error in (no error)"=w457) -> ("error out"=w452:errorcluster)  [unwired: 9 in, 1 out]
        n182 = control-ref of="instr param table"() -> (w454:refnum<vi>)
        n183 = property class="Tbl (strict)"(reference=w454, error in=w452) -> ("Value"=w453:string[][])  [unwired: 2 out]
        n184 = call "DataXML saveXMLProcess.vi"("addTagName"="System" ("add tag name"), "newData"=w453) -> ("error out"=w451:errorcluster)  [unwired: 9 in]
        n185 = call "_PC_Err write_error_message.vi"("show msg( T )"=FALSE, "error in"=w451) -> ("error out"=w458:errorcluster)  [unwired: 9 in]
        n186 = call <vilib>:"Unset Busy.vi"("error in (no error)"=w458) -> ("error out"=w456:errorcluster)  [unwired: 10 in]
      }
      frame "exportInstr" {
        n187 = call <vilib>:"Set Busy.vi"("error in (no error)"=w471) -> ("error out"=w474:errorcluster)  [unwired: 9 in, 1 out]
        n188 = Variant To Data(error in=w474, type=string[][] [] ("NewVal"), Variant=w472) -> (data=w475:string[][], error out=w465:errorcluster)
        n189 = call <vilib>:"Application Directory.vi"() -> ("Application Directory"=w469:path)
        n190 = call "File Dialog4"("start path"=w469, "prompt"="Export Instrument Parameter", "default name"="Param", "error in"=w465, "pattern (all files)"="*.instr") -> ("selected path"=w463:path, "exists"=w461:bool, "cancelled"=w462:bool, "error out"=w464:errorcluster)  [unwired: 7 in]
        n191 = case shown="No Error" w464 {
          selector: w464 -> [_ w494]
          tunnel: w475 -> [w476 _]
          tunnel: [_ w495] -> w470
          tunnel: w463 -> [w479 _]
          tunnel: w462 -> [w478 _]
          tunnel: w461 -> [w477 _]
          frame No Error {
            n192 = case shown="False" w478 {
              tunnel: w479 -> [w482 _]
              tunnel: w477 -> [w483 _]
              tunnel: w476 -> [w480 _]
              frame False {
                n193 = case shown="True" w483 {
                  tunnel: [TRUE w490] -> w481
                  frame False {
                  }
                  frame True {
                    n194 = Two Button Dialog(message="Do you want to overwrite this file ?", 1:"No" ("F button name (\"Cancel\")"), 2:"Yes" ("T button name (\"OK\")")) -> (T button?=w490:bool)
                  }
                }
                n195 = case shown="False" w481 {
                  tunnel: w482 -> [_ w486]
                  tunnel: w480 -> [_ w488]
                  frame False {
                  }
                  frame True {
                    n196 = call "DataXML saveXMLProcess.vi"("addTagName"="System" ("add tag name"), "dataType"=DataXML_dataType."UserDefined", "appended path"=w486, "rootNodeName"="Instrument", "newData"=w488) -> ()  [unwired: 6 in, 1 out]
                  }
                }
              }
              frame True {
              }
            }
          }
          frame Error {
            n197 = call "_PC_Err write_error_message.vi"("show msg( T )"=FALSE, "error in"=w494) -> ("error out"=w495:errorcluster)  [unwired: 9 in]
          }
        }
        n198 = call <vilib>:"Unset Busy.vi"("error in (no error)"=w470) -> ("error out"=w460:errorcluster)  [unwired: 10 in]
      }
      frame "importInstr" {
        n199 = call <vilib>:"Application Directory.vi"() -> ("Application Directory"=w508:path)
        n200 = call <vilib>:"Set Busy.vi"("error in (no error)"=w499) -> ("error out"=w501:errorcluster)  [unwired: 9 in, 1 out]
        n201 = control-ref of="instr param table"() -> (w500:refnum<vi>)
        n202 = call "File Dialog5"("start path"=w508, "prompt"="Import Instrument Parameter", "default name"="Param", "error in"=w501, "pattern (all files)"="*.instr") -> ("selected path"=w503:path, "cancelled"=w502:bool, "error out"=w504:errorcluster)  [unwired: 7 in, 1 out]
        n203 = case shown="No Error" w504 {
          selector: w504 -> [w511 w534]
          tunnel: w503 -> [w513 _]
          tunnel: w502 -> [w512 _]
          tunnel: w500 -> [w510 _]
          tunnel: [w509 w533] -> w498
          frame No Error {
            n204 = case shown="False" w512 {
              tunnel: w513 -> [w529 _]
              tunnel: w511 -> [w528 w532]
              tunnel: w510 -> [w520 _]
              tunnel: [w516 w532] -> w509
              frame False {
                n205 = call "DataXML loadXmlProcess.vi"("target name"="System", "level"=u8 1, "error in (no error)"=w528, "xml_data_path"=w529) -> ("error IO"=w519:errorcluster, "value"=w525:string[], "name"=w526:string[])  [unwired: 4 in, 1 out]
                n206 = Build Array(w526, w525) -> (w527:string[][])
                n207 = Transpose 2D Array(2D array=w527) -> (transposed array=w514:string[][])
                n208 = property class="Tbl (strict)"(reference=w520, error in=w519, "Value"=w514) -> (reference out=w524:refnum<vi>, error out=w523:errorcluster)
                n209 = property class="Tbl (strict)"(reference=w524, error in=w523, "Active Cell"=T4 {"Row"=-2, "Column"=-2} ("Active Cell:Active Cell")) -> (reference out=w522:refnum<vi>, error out=w521:errorcluster)
                n210 = call "DataXML saveXMLProcess.vi"("addTagName"="System" ("add tag name"), "newData"=w514) -> ()  [unwired: 9 in, 1 out]
                n211 = property class="Tbl (strict)"(reference=w522, error in=w521, "Cell BG Color"=u32 16448250) -> (error out=w516:errorcluster)  [unwired: 1 out]
              }
              frame True {
              }
            }
          }
          frame Error {
            n212 = call "_PC_Err write_error_message.vi"("show msg( T )"=FALSE, "error in"=w534) -> ("error out"=w533:errorcluster)  [unwired: 9 in]
          }
        }
        n213 = call <vilib>:"Unset Busy.vi"("error in (no error)"=w498) -> ("error out"=w497:errorcluster)  [unwired: 10 in]
      }
      frame "help" {
        n214 = call "_PC_Pub openHelperHtml.vi"("error in (no error)"=w538, "procType"=enum16{"none", "MSProcess", "SignalProcess"}."MSProcess") -> ("error out"=w537:errorcluster)  [unwired: 1 out]
        n215 = call "_PC_Err write_error_message.vi"("show msg( T )"=TRUE, "error in"=w537) -> ()  [unwired: 9 in, 1 out]
      }
      frame "close" {
        n216 = Variant To Data(error in=w540, type="", Variant=w554) -> (data=w550:string, error out=w552:errorcluster)
        n217 = Empty String/Path?(string/path=w550) -> (empty?=w551:bool)
        n218 = case shown="False" w551 {
          tunnel: w552 -> [w559 w562]
          tunnel: w550 -> [w561 _]
          tunnel: [w560 _] -> _
          tunnel: [w559 w562] -> w549
          frame False {
            n219 = One Button Dialog(message=w561) -> (true=w560:bool)  [unwired: 1 in]
          }
          frame True {
          }
        }
        n220 = call <vilib>:"Clear Errors.vi"("error in (no error)"=w549) -> ("error out"=w547:errorcluster)  [unwired: 5 in, 1 out]
        n221 = call "_PC_Tab_CaptureData.vi"("Function"=enum16{"Init", "Get Data", "Update", "Close"}."Update", "error in (no error)"=w547) -> ("error out"=w545:errorcluster)  [unwired: 9 in]
        n222 = call "_PC_Err write_error_message.vi"("show msg( T )"=FALSE, "error in"=w545) -> ("error out"=w542:errorcluster)  [unwired: 9 in]
        n223 = control-ref of="stop"() -> (w543:refnum<vi>)
        n224 = property class="Bool (strict)"(reference=w543, error in=w542, "Val(Sgnl)"=TRUE ("Value (Signaling)")) -> (error out=w541:errorcluster)  [unwired: 1 out]
        n225 = control-ref of="This VI"() -> (w557:refnum<vi>)
        n226 = property class="VI"(reference=w557, error in=w541, "FP:Transparency"=u8 100 ("Front Panel Window:Transparency")) -> (error out=w555:errorcluster)  [unwired: 1 out]
      }
    }
  }
  "error out" <- w49
  n227 = while {
    tunnel: w2 -> [w569]
    tunnel: w1 -> [w568]
    tunnel: "script" -> [w567]
    tunnel: w15 -> [w566]
    tunnel: w11 -> [w565]
    tunnel: T1."Disabled and Grayed Out" ("Disabled") -> [w564]
    tunnel: w9 -> [w563]
    stop <- w570 stop-if-true
    # "Recipe Function"
    n228 = event shown="[1] \"script\": Key Down?" {
      selector: _ -> [_ _ _]
      dyn-events: _ -> [_ _ _]
      timeout: _ -> [_ _ _]
      tunnel: [_ _ w589] -> w570
      tunnel: w569 -> [_ w582 w586]
      tunnel: w568 -> [_ w581 w587]
      tunnel: w567 -> [_ _ w588]
      tunnel: w566 -> [_ w576 _]
      tunnel: w565 -> [_ w575 _]
      tunnel: w564 -> [_ w573 _]
      tunnel: w563 -> [_ w574 _]
      event Timeout {
        n229 = event-data() -> ()  [unwired: 1 in, 1 out]
      }
      event "script": Key Down? {
        n230 = event-data() -> ("PlatMods.Ctrl"=w571:bool, "VKey"=w580:T12, "Char"=w579:i16)  [unwired: 1 in]
        n231 = property class="Bool"(reference=w574, "DisabledEnum"=w573) -> ()  [unwired: 1 in, 2 out]
        n232 = property class="Bool"(reference=w575, "DisabledEnum"=w573) -> ()  [unwired: 1 in, 2 out]
        n233 = control-ref of="searchText"() -> (w572:refnum<vi>)
        n234 = call "winForms keyDownResponse.vi"("searchString"=w572, "editorType"=w576, "Ctrl"=w571, "error in (no error)"=w581, "Char"=w579, "VKey"=w580, "scintillaRefNum"=w582) -> ("error out"=w577:errorcluster, "Discard?"=w578:bool)  [unwired: 3 in]
        n235 = call "_PC_Err write_error_message.vi"("error in"=w577) -> ()  [unwired: 10 in, 1 out]
        n236 = event-data("Discard?"=w578) -> ()  [unwired: 1 in, 1 out]
      }
      event "stop": Value Change {
        n237 = event-data() -> ("NewVal"=w589:bool)  [unwired: 1 in]
        n238 = invoke class="Scintilla" method="ClearAll"(reference=w586, error in=w587) -> (reference out=w584:refnum<k24>, error out=w585:errorcluster)  [unwired: 1 in, 1 out]
        n239 = Close Reference(reference=w584, error in (no error)=w585) -> (error out=w583:errorcluster)
        n240 = Close Reference(reference=w588, error in (no error)=w583) -> ()  [unwired: 1 out]
      }
    }
  }
  n241 = while {
    tunnel: w32 -> [w595]
    tunnel: w31 -> [w594]
    shift-right: [w593] -> _
    shift-left: 0 ("Position") -> [w592]
    shift-right: [w591] -> _
    shift-left: 0 -> [w590]
    tunnel: w17 -> [_]
    stop <- w596 stop-if-true
    # "Tab Resize Function"
    n242 = event shown="[1] \"param_pane\": Pane Size" {
      selector: _ -> [_ _ _]
      dyn-events: _ -> [_ _ _]
      timeout: _ -> [_ _ _]
      tunnel: [_ w597 w617] -> w596
      tunnel: w595 -> [_ w606 _]
      tunnel: w594 -> [_ w604 _]
      tunnel: [_ w605 _] -> w593
      tunnel: w592 -> [_ w600 _]
      tunnel: [_ w599 _] -> w591
      tunnel: w590 -> [_ w598 _]
      event Timeout {
        n243 = event-data() -> ()  [unwired: 1 in, 3 out]
      }
      event Pane Size {
        n244 = event-data() -> ()  [unwired: 1 in, 1 out]
        n245 = property class="Splitter"(reference=w604) -> (reference out=w603:refnum<vi>, "Position"=w602:i32)  [unwired: 1 in, 1 out]
        n246 = Equal?(x=w602, y=w600) -> (x = y?=w601:bool)
        n247 = case shown="True" w601 {
          tunnel: w606 -> [w607 _]
          tunnel: w603 -> [w610 _]
          tunnel: [w608 w616] -> w605
          tunnel: w600 -> [_ w616]
          tunnel: [_ w614] -> w599
          tunnel: w598 -> [_ w615]
          tunnel: [_ w612] -> w597
          frame False {
            n248 = property class="Splitter"(reference=w610) -> (reference out=w609:refnum<vi>, "Position"=w608:i32)  [unwired: 1 in, 1 out]
            n249 = call "recipeScript resizeParamTab.vi"("dialogueTopSpl"=w609, "Parameter Tab"=w607) -> ("error out"=w611:errorcluster)  [unwired: 9 in]
            n250 = call "_PC_Err write_error_message.vi"("error in"=w611) -> ()  [unwired: 10 in, 1 out]
          }
          frame True {
            n251 = Increment(x=w615) -> (x+1=w614:i32)
            n252 = Greater?(x=w614, y=30) -> (0:w612:bool)
          }
        }
      }
      event "stop": Value Change {
        n253 = event-data() -> ("NewVal"=w617:bool)  [unwired: 1 in]
      }
    }
  }
  n254 = while {
    tunnel: w61 -> [w620]
    tunnel: w48 -> [w619]
    stop <- w618 stop-if-true
    n255 = event shown="[7] \"checkScript\": Value Change" {
      selector: _ -> [_ _ _ _ _ _ _ _ _ _ _ _ _ _ _ _ _ _]
      dyn-events: _ -> [_ _ _ _ _ _ _ _ _ _ _ _ _ _ _ _ _ _]
      timeout: _ -> [_ _ _ _ _ _ _ _ _ _ _ _ _ _ _ _ _ _]
      tunnel: w620 -> [_ _ _ w643 w662 w691 w719 w732 w738 w741 _ _ _ _ w800 w807 w820 w829]
      tunnel: w619 -> [_ _ _ w639 w651 w688 w714 w727 w735 w740 _ _ _ w795 w799 w804 w817 w828]
      tunnel: [_ _ _ _ _ _ _ _ _ _ _ _ _ _ _ _ _ TRUE] -> w618
      event Timeout {
        n256 = event-data() -> ()  [unwired: 1 in, 3 out]
      }
      event Mouse Move {
        n257 = event-data() -> ()  [unwired: 1 in, 5 out]
        n258 = call "_PC_Pub ctrlRegistry.vi"("type"=enum16{"None", "Write", "Read"}."Write", "function"=RegistyFunc."ExeStatu", "write value"=u32 1) -> ()  [unwired: 5 in, 4 out]
      }
      event "file path": Value Change {
        n259 = event-data() -> ("CtlRef"=w626:refnum<vi>, "OldVal"=w628:string, "NewVal"=w627:string)  [unwired: 1 in]
        n260 = String To Path(string=w627) -> (path=w631:path)
        n261 = Not A Number/Path/Refnum?(number/path/refnum=w631) -> (NaN/Path/Refnum?=w630:bool)
        n262 = Empty String/Path?(string/path=w631) -> (empty?=w629:bool)
        n263 = Or(x=w630, y=w629) -> (x .or. y?=w624:bool)
        n264 = Select(t=w628, s=w624, f=w627) -> (s? t:f=w625:string)
        n265 = case shown="True" w624 {
          frame False {
          }
          frame True {
            n266 = One Button Dialog(message="Invalid path") -> ()  [unwired: 1 in, 1 out]
          }
        }
        n267 = property class="Str"(reference=w626, "Value"=w625) -> ()  [unwired: 1 in, 2 out]
      }
      event "SaveScript": Value Change {
        n268 = event-data() -> ("CtlRef"=w644:refnum<vi>)  [unwired: 1 in]
        n269 = property class="Bool"(reference=w644, error in=w639, "DisabledEnum"=T1."Disabled" ("Disabled")) -> (reference out=w641:refnum<vi>, error out=w637:errorcluster)
        n270 = call "_PC_Pub_WaitCmd.vi"("milliseconds to wait"=u32 200, "error in (no error)"=w637) -> ("error out"=w636:errorcluster)  [unwired: 9 in]
        n271 = call "_QMH_Enqueue.vi"("error in (no error)"=w636, "Msg"="saveScript", "QMH in"=w643) -> ("error out"=w634:errorcluster)  [unwired: 7 in, 1 out]
        n272 = call "_PC_Pub_WaitCmd.vi"("milliseconds to wait"=u32 500, "error in (no error)"=w634) -> ("error out"=w633:errorcluster)  [unwired: 9 in]
        n273 = property class="Bool"(reference=w641, error in=w633, "DisabledEnum"=T1."Enabled" ("Disabled")) -> ()  [unwired: 2 out]
      }
      event "open script": Value Change; "file path": Mouse Up {
        n274 = event-data() -> ()  [unwired: 1 in, 1 out]
        n275 = control-ref of="open script"() -> (w652:refnum<vi>)
        n276 = property class="Bool"(reference=w652, error in=w651, "DisabledEnum"=T1."Disabled" ("Disabled")) -> (reference out=w658:refnum<vi>, error out=w650:errorcluster)
        n277 = control-ref of="file path"() -> (w660:refnum<vi>)
        n278 = property class="Str"(reference=w660, error in=w650) -> ("Value"=w661:string)  [unwired: 2 out]
        n279 = String To Path(string=w661) -> (path=w646:path)
        n280 = call "File Dialog"("start path"=w646, "prompt"="Open Script", "error in"=w650, "pattern (all files)"="*.arp" ("extension name")) -> ("selected path"=w663:path, "exists"=w664:bool, "cancelled"=w665:bool, "error out"=w648:errorcluster)  [unwired: 8 in]
        n281 = call "_PC_Pub_WaitCmd.vi"("milliseconds to wait"=u32 200, "error in (no error)"=w648) -> ("error out"=w647:errorcluster)  [unwired: 9 in]
        n282 = case shown="False" w665 {
          tunnel: w664 -> [w668 _]
          tunnel: w663 -> [w667 _]
          tunnel: w662 -> [w670 _]
          tunnel: w647 -> [w669 w679]
          tunnel: [w666 w678] -> w654
          frame False {
            n283 = case shown="True" w668 {
              tunnel: w670 -> [_ w674]
              tunnel: w669 -> [w672 w673]
              tunnel: w667 -> [_ w676]
              tunnel: [w671 w675] -> w666
              frame False {
                n284 = call <vilib>:"Clear Errors.vi"("error in (no error)"=w672) -> ("error out"=w671:errorcluster)  [unwired: 5 in, 1 out]
              }
              frame True {
                n285 = call "_QMH_Enqueue.vi"("error in (no error)"=w673, "Data"=w676, "Msg"="openFile", "QMH in"=w674) -> ("error out"=w675:errorcluster)  [unwired: 6 in, 1 out]
              }
            }
          }
          frame True {
            n286 = call <vilib>:"Clear Errors.vi"("error in (no error)"=w679) -> ("error out"=w678:errorcluster)  [unwired: 5 in, 1 out]
          }
        }
        n287 = call "_PC_Err write_error_message.vi"("error in"=w654) -> ("error out"=w653:errorcluster)  [unwired: 10 in]
        n288 = property class="Bool"(reference=w658, error in=w653, "DisabledEnum"=T1."Enabled" ("Disabled")) -> ()  [unwired: 2 out]
      }
      event "SaveScript_new": Value Change {
        n289 = event-data() -> ("CtlRef"=w698:refnum<vi>)  [unwired: 1 in]
        n290 = property class="Bool"(reference=w698, error in=w688, "DisabledEnum"=T1."Disabled" ("Disabled")) -> (reference out=w697:refnum<vi>, error out=w690:errorcluster)
        n291 = control-ref of="file path"() -> (w689:refnum<vi>)
        n292 = property class="Str"(reference=w689, error in=w688) -> ("Value"=w687:string)  [unwired: 2 out]
        n293 = String To Path(string=w687) -> (path=w680:path)
        n294 = call "File Dialog3"("start path"=w680, "prompt"="Select script file ,  or create new file", "error in"=w690, "pattern (all files)"="*.arp" ("extension name")) -> ("selected path"=w694:path, "cancelled"=w695:bool, "error out"=w685:errorcluster)  [unwired: 8 in, 1 out]
        n295 = call "_PC_Pub_WaitCmd.vi"("milliseconds to wait"=u32 200, "error in (no error)"=w685) -> ("error out"=w684:errorcluster)  [unwired: 9 in]
        n296 = case shown="False" w695 {
          tunnel: w694 -> [w702 _]
          tunnel: w691 -> [w701 _]
          tunnel: w684 -> [w700 w706]
          tunnel: [w703 w705] -> w682
          frame False {
            n297 = call "_QMH_Enqueue.vi"("error in (no error)"=w700, "Data"=w702, "Msg"="saveScript", "QMH in"=w701) -> ("error out"=w703:errorcluster)  [unwired: 6 in, 1 out]
          }
          frame True {
            n298 = call <vilib>:"Clear Errors.vi"("error in (no error)"=w706) -> ("error out"=w705:errorcluster)  [unwired: 5 in, 1 out]
          }
        }
        n299 = call "_PC_Pub_WaitCmd.vi"("milliseconds to wait"=u32 500, "error in (no error)"=w682) -> ("error out"=w681:errorcluster)  [unwired: 9 in]
        n300 = property class="Bool"(reference=w697, error in=w681, "DisabledEnum"=T1."Enabled" ("Disabled")) -> ()  [unwired: 2 out]
      }
      event "applyScript": Value Change {
        n301 = event-data() -> ("CtlRef"=w716:refnum<vi>)  [unwired: 1 in]
        n302 = property class="Bool"(reference=w716, error in=w714, "DisabledEnum"=T1."Disabled" ("Disabled")) -> (reference out=w713:refnum<vi>, error out=w711:errorcluster)
        n303 = call "_PC_Pub_WaitCmd.vi"("milliseconds to wait"=u32 200, "error in (no error)"=w711) -> ("error out"=w710:errorcluster)  [unwired: 9 in]
        n304 = call "_QMH_Enqueue.vi"("error in (no error)"=w710, "Msg"="applyPy", "QMH in"=w719) -> ("error out"=w708:errorcluster)  [unwired: 7 in, 1 out]
        n305 = call "_PC_Pub_WaitCmd.vi"("milliseconds to wait"=u32 500, "error in (no error)"=w708) -> ("error out"=w707:errorcluster)  [unwired: 9 in]
        n306 = property class="Bool"(reference=w713, error in=w707, "DisabledEnum"=T1."Enabled" ("Disabled")) -> ()  [unwired: 2 out]
      }
      event "checkScript": Value Change {
        n307 = event-data() -> ("CtlRef"=w729:refnum<vi>)  [unwired: 1 in]
        n308 = property class="Bool"(reference=w729, error in=w727, "DisabledEnum"=T1."Disabled" ("Disabled")) -> (reference out=w726:refnum<vi>, error out=w724:errorcluster)
        n309 = call "_PC_Pub_WaitCmd.vi"("milliseconds to wait"=u32 200, "error in (no error)"=w724) -> ("error out"=w723:errorcluster)  [unwired: 9 in]
        n310 = call "_QMH_Enqueue.vi"("error in (no error)"=w723, "Msg"="checkPy", "QMH in"=w732) -> ("error out"=w721:errorcluster)  [unwired: 7 in, 1 out]
        n311 = call "_PC_Pub_WaitCmd.vi"("milliseconds to wait"=u32 500, "error in (no error)"=w721) -> ("error out"=w720:errorcluster)  [unwired: 9 in]
        n312 = property class="Bool"(reference=w726, error in=w720, "DisabledEnum"=T1."Enabled" ("Disabled")) -> ()  [unwired: 2 out]
      }
      event "save_method": Value Change {
        n313 = event-data() -> ()  [unwired: 1 in, 1 out]
        n314 = call "_PC_Pub_WaitCmd.vi"("milliseconds to wait"=u32 200, "error in (no error)"=w735) -> ("error out"=w734:errorcluster)  [unwired: 9 in]
        n315 = call "_QMH_Enqueue.vi"("error in (no error)"=w734, "Msg"="saveMthd", "QMH in"=w738) -> ("error out"=w733:errorcluster)  [unwired: 7 in, 1 out]
        n316 = call "_PC_Pub_WaitCmd.vi"("milliseconds to wait"=u32 500, "error in (no error)"=w733) -> ()  [unwired: 9 in, 1 out]
      }
      event "help": Value Change {
        n317 = event-data() -> ()  [unwired: 1 in, 1 out]
        n318 = call "_PC_Pub_WaitCmd.vi"("milliseconds to wait"=u32 200, "error in (no error)"=w740) -> ("error out"=w743:errorcluster)  [unwired: 9 in]
        n319 = call "_QMH_Enqueue.vi"("error in (no error)"=w743, "Msg"="help", "QMH in"=w741) -> ("error out"=w742:errorcluster)  [unwired: 7 in, 1 out]
        n320 = call "_PC_Pub_WaitCmd.vi"("milliseconds to wait"=u32 500, "error in (no error)"=w742) -> ()  [unwired: 9 in, 1 out]
      }
      event "instr param table": Mouse Down? {
        n321 = event-data() -> ("CtlRef"=w763:refnum<vi>, "Coords"=w762:T14)  [unwired: 1 in]
        n322 = invoke class="Tbl (strict)" method="Point To Row Column"(reference=w763, "Point"=w762) -> (reference out=w760:refnum<vi>, error out=w759:errorcluster, "CellPosition"=w761:T4)  [unwired: 4 in, 3 out]
        n323 = property class="Tbl (strict)"(reference=w760, error in=w759) -> (reference out=w753:refnum<vi>, error out=w751:errorcluster, "Value"=w758:string[][])
        n324 = Array Size(array=w758) -> (size(s)=w757:i32[])
        n325 = Unbundle By Name(w761) -> ("Row"=w755:i32, "Column"=w750:i32)
        n326 = Index Array(array=w757, index=0) -> (element=w754:i32)
        n327 = Greater Or Equal?(x=w755, y=w754) -> (x >= y?=w749:bool)
        n328 = Equal To 0?(x=w750) -> (x = 0?=w748:bool)
        n329 = property class="Tbl (strict)"(reference=w753, error in=w751, "Key Focus"=FALSE) -> ()  [unwired: 2 out]
        n330 = Or(x=w749, y=w748) -> (x .or. y?=w747:bool)
        n331 = event-data("Discard?"=w747) -> ()  [unwired: 1 in, 1 out]
      }
      event "user param table": Mouse Down? {
        n332 = event-data() -> ("CtlRef"=w777:refnum<vi>, "Coords"=w776:T14)  [unwired: 1 in]
        n333 = invoke class="Tbl (strict)" method="Point To Row Column"(reference=w777, "Point"=w776) -> (reference out=w774:refnum<vi>, error out=w773:errorcluster, "CellPosition"=w775:T4)  [unwired: 4 in, 3 out]
        n334 = property class="Tbl (strict)"(reference=w774, error in=w773) -> (reference out=w767:refnum<vi>, error out=w765:errorcluster, "Value"=w772:string[][])
        n335 = Array Size(array=w772) -> (size(s)=w771:i32[])
        n336 = Unbundle By Name(w775) -> ("Row"=w769:i32)
        n337 = Index Array(array=w771, index=0) -> (element=w768:i32)
        n338 = Greater?(x=w769, y=w768) -> (0:w764:bool)
        n339 = property class="Tbl (strict)"(reference=w767, error in=w765, "Key Focus"=FALSE) -> ()  [unwired: 2 out]
        n340 = event-data("Discard?"=w764) -> ()  [unwired: 1 in, 1 out]
      }
      event "instr param table", "user param table": Key Down? {
        n341 = event-data() -> ("CtlRef"=w779:refnum<vi>, "Char"=w782:i16, "VKey"=w781:T12)  [unwired: 1 in]
        n342 = case shown="\"Return\"" w781 {
          tunnel: w782 -> [_ w789 _]
          tunnel: [_ w787 TRUE] -> w780
          frame "Escape", Default {
          }
          frame "ASCII" {
            n343 = Equal?(x=i16 9, y=w789) -> (x = y?=w787:bool)
          }
          frame "Return" {
          }
        }
        n344 = case shown="True" w780 {
          selector: w780 -> [w783 w786]
          tunnel: [w783 w786] -> w778
          tunnel: w779 -> [_ w785]
          frame False {
          }
          frame True {
            n345 = property class="Tbl (strict)"(reference=w785, "Key Focus"=FALSE) -> ()  [unwired: 1 in, 2 out]
          }
        }
        n346 = event-data("Discard?"=w778) -> ()  [unwired: 1 in, 1 out]
      }
      event "instr param table": Shortcut Menu Activation? {
        n347 = event-data() -> ("MenuRef"=w796:refnum<k9>)  [unwired: 1 in]
        n348 = Delete Menu Items(6:w795, 9:w796) -> (0:w793:errorcluster, 3:w794:refnum<k9>)  [unwired: 2 in]
        n349 = Insert Menu Items(6:w793, 7:string[] ["importInstr", "exportInstr"] ("item tags"), 8:string[] ["Import Parameter", "Export Parameter"] ("item names"), 9:w794) -> ()  [unwired: 2 in, 3 out]
        n350 = event-data() -> ()  [unwired: 2 in, 1 out]
      }
      event "instr param table": Shortcut Menu Selection (User) {
        n351 = event-data() -> ("ItemTag"=w801:string, "CtlRef"=w798:refnum<vi>)  [unwired: 1 in]
        n352 = property class="Tbl (strict)"(reference=w798) -> ("Value"=w797:string[][])  [unwired: 1 in, 2 out]
        n353 = call "_QMH_Enqueue.vi"("error in (no error)"=w799, "Data"=w797, "Msg"=w801, "QMH in"=w800) -> ()  [unwired: 6 in, 2 out]
      }
      event "user param table": Value Change {
        n354 = event-data() -> ("CtlRef"=w806:refnum<vi>, "NewVal"=w805:string[][])  [unwired: 1 in]
        n355 = call <vilib>:"Set Busy.vi"("error in (no error)"=w804) -> ("error out"=w803:errorcluster)  [unwired: 9 in, 1 out]
        n356 = call "recipeScript checkTableParam.vi"("error in (no error)"=w803, "newVal"=w805, "tableRefNum"=w806) -> ("error out"=w809:errorcluster, "valid"=w808:bool)  [unwired: 7 in]
        n357 = case shown="False" w808 {
          tunnel: w807 -> [_ w813]
          tunnel: w809 -> [w810 w812]
          tunnel: [w810 w811] -> w802
          frame False {
          }
          frame True {
            n358 = call "_QMH_Enqueue.vi"("error in (no error)"=w812, "Msg"="userParamUpd", "QMH in"=w813) -> ("error out"=w811:errorcluster)  [unwired: 7 in, 1 out]
          }
        }
        n359 = call <vilib>:"Unset Busy.vi"("error in (no error)"=w802) -> ()  [unwired: 10 in, 1 out]
      }
      event "instr param table": Value Change {
        n360 = event-data() -> ("CtlRef"=w819:refnum<vi>, "NewVal"=w818:string[][])  [unwired: 1 in]
        n361 = call <vilib>:"Set Busy.vi"("error in (no error)"=w817) -> ("error out"=w816:errorcluster)  [unwired: 9 in, 1 out]
        n362 = call "recipeScript checkTableParam.vi"("error in (no error)"=w816, "newVal"=w818, "tableRefNum"=w819) -> ("error out"=w822:errorcluster, "valid"=w821:bool)  [unwired: 7 in]
        n363 = case shown="True" w821 {
          tunnel: w820 -> [_ w826]
          tunnel: w822 -> [w823 w825]
          tunnel: [w823 w824] -> w815
          frame False {
          }
          frame True {
            n364 = call "_QMH_Enqueue.vi"("error in (no error)"=w825, "Msg"="instrParamUpd", "QMH in"=w826) -> ("error out"=w824:errorcluster)  [unwired: 7 in, 1 out]
          }
        }
        n365 = call <vilib>:"Unset Busy.vi"("error in (no error)"=w815) -> ()  [unwired: 10 in, 1 out]
      }
      event Panel Close {
        n366 = event-data() -> ()  [unwired: 1 in, 1 out]
        n367 = call "_QMH_Enqueue.vi"("error in (no error)"=w828, "Msg"="close", "QMH in"=w829) -> ()  [unwired: 7 in, 2 out]
      }
    }
  }
